vi "delta T.vi"(11 "Tranfer speed":T1) -> (3 "dt":dbl=1e-06 format="%#_13g")   [LabVIEW 2018]
uses:
  controls/host_transfer_speed.ctl
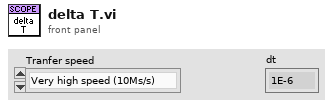
[diagram p1: front panel]
types:
  T1 = typedef "host_transfer_speed.ctl" = enum16{"Very high speed (10Ms/s)", "High speed (1Ms/s)", "Low speed (50kS/s)", "Ultra low speed (20kS/s)"}
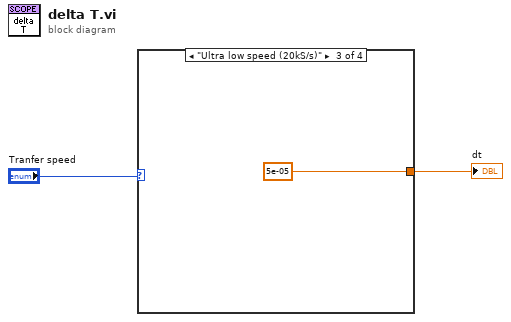
[diagram p0: block diagram]
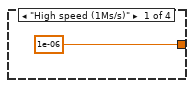
[diagram p2: hidden frame]
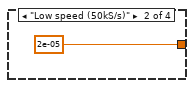
[diagram p3: hidden frame]
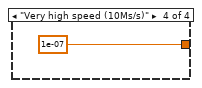
[diagram p4: hidden frame]
diagram:
  n1 = case shown="\"Ultra low speed (20kS/s)\"" "Tranfer speed" {
    tunnel: [1e-06 2e-05 5e-05 1e-07] -> w1
    frame "High speed (1Ms/s)" {
    }
    frame "Low speed (50kS/s)" {
    }
    frame "Ultra low speed (20kS/s)" {
    }
    frame "Very high speed (10Ms/s)" {
    }
  }
  "dt" <- w1
